vi "MemoryInitialize.vi"(8 "error in (no error)":errorcluster) -> (0 "error out":errorcluster)   [LabVIEW 2015]
uses:
  <vilib>/userdefined/High Color/IMAQdx.ctl
  [Global]CamNumber.vi
  [Global]ForCalCalculaton.vi
  [Global] ExtractedAnalizedImage.vi
  [Global] OperatorsImageTemplate2.vi
  [Global] ExtractedProcessImage.vi
  [Global] Coord.vi
  [Global] ExtractedImage.vi
  [Global] CameraSessionArray.vi
  [Global] CameraNameArray.vi
  [Global] Image.vi
  [Global] Image Overlay.vi
  [Global]Script Number.vi
  [Global]PatternMatchNumber.vi
  [Global] Template.vi
  [Global]SeqNumber.vi
  [Global]CalTemp.vi
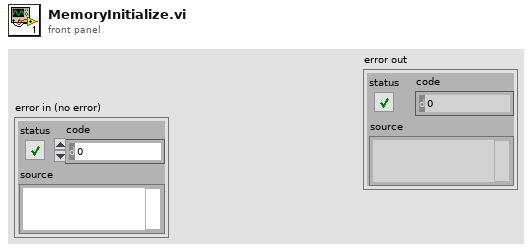
[diagram p1: front panel]
types:
  T1 = typedef "IMAQdx.ctl" = refnum<k21>
  T2 = typedef "IMAQ Image.ctl" = refnum<image>
  T3 = cluster{"Image Name":string, cluster{"Image Name":string, "New Image":T2}[]}
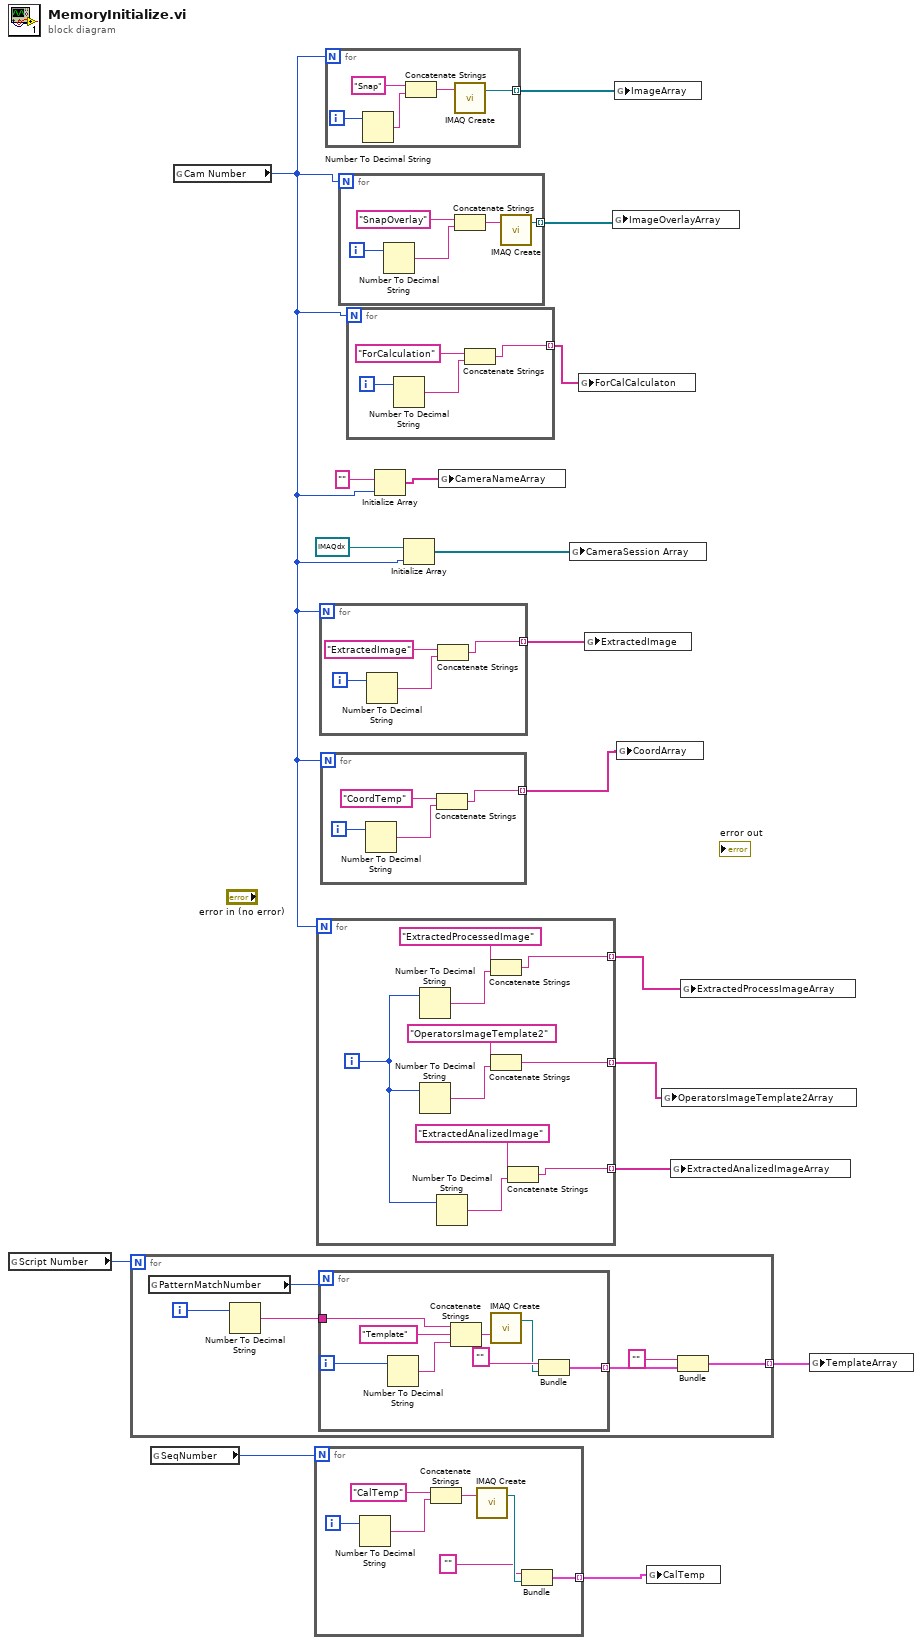
[diagram p0: block diagram]
diagram:
  n1 = global read "[Global]Script Number.vi" "Script Number"() -> (w3:i32)
  n2 = for {
    N: w3 -> [_]
    tunnel: [w18] -> w2 mode=indexing
    i -> [w20]
    n3 = global read "[Global]PatternMatchNumber.vi" "PatternMatchNumber"() -> (w21:i32)
    n4 = Number To Decimal String(number=w20) -> (decimal integer string=w19:string)  [unwired: 1 in]
    n5 = for {
      N: w21 -> [_]
      tunnel: [w29] -> w23 mode=indexing
      tunnel: w19 -> [w24]
      i -> [w27]
      n6 = Number To Decimal String(number=w27) -> (decimal integer string=w30:string)  [unwired: 1 in]
      n7 = Concatenate Strings(w24, "Template" ("Image Name"), w30) -> (w26:string)
      n8 = call "IMAQ Create"("Image Name"=w26) -> ("New Image"=w25:T2)  [unwired: 3 in, 2 out]
      n9 = Bundle("Image Name"="", "New Image"=w25) -> (w29:cluster{"Image Name":string, "New Image":T2})  [unwired: 1 in]
    }
    n10 = Bundle("Image Name"="", w23) -> (w18:T3)  [unwired: 1 in]
  }
  n11 = global read "[Global]SeqNumber.vi" "SeqNumber"() -> (w7:i32)
  n12 = global read "[Global]CamNumber.vi" "Cam Number"() -> (w5:i32)
  n13 = for {
    N: w7 -> [_]
    tunnel: [w32] -> w6 mode=indexing
    i -> [w37]
    n14 = Number To Decimal String(number=w37) -> (decimal integer string=w36:string)  [unwired: 1 in]
    n15 = Concatenate Strings("CalTemp" ("Image Name"), w36) -> (w35:string)
    n16 = call "IMAQ Create"("Image Name"=w35) -> ("New Image"=w34:T2)  [unwired: 3 in, 2 out]
    n17 = Bundle("Image Name"="", "New Image"=w34) -> (w32:cluster{"Image Name":string, "New Image":T2})  [unwired: 1 in]
  }
  n18 = for {
    N: w5 -> [_]
    tunnel: [w46] -> w10 mode=indexing
    tunnel: [w43] -> w9 mode=indexing
    tunnel: [w40] -> w8 mode=indexing
    i -> [w39]
    n19 = Number To Decimal String(number=w39) -> (decimal integer string=w47:string)  [unwired: 1 in]
    n20 = Number To Decimal String(number=w39) -> (decimal integer string=w45:string)  [unwired: 1 in]
    n21 = Number To Decimal String(number=w39) -> (decimal integer string=w41:string)  [unwired: 1 in]
    n22 = Concatenate Strings("ExtractedProcessedImage" ("Image Name"), w47) -> (w46:string)
    n23 = Concatenate Strings("OperatorsImageTemplate2" ("Image Name"), w45) -> (w43:string)
    n24 = Concatenate Strings("ExtractedAnalizedImage" ("Image Name"), w41) -> (w40:string)
  }
  n25 = for {
    N: w5 -> [_]
    tunnel: [w49] -> w11 mode=indexing
    i -> [w51]
    n26 = Number To Decimal String(number=w51) -> (decimal integer string=w50:string)  [unwired: 1 in]
    n27 = Concatenate Strings("ExtractedImage" ("Image Name"), w50) -> (w49:string)
  }
  n28 = for {
    N: w5 -> [_]
    tunnel: [w53] -> w1 mode=indexing
    i -> [w55]
    n29 = Number To Decimal String(number=w55) -> (decimal integer string=w54:string)  [unwired: 1 in]
    n30 = Concatenate Strings("CoordTemp" ("Image Name"), w54) -> (w53:string)
  }
  n31 = for {
    N: w5 -> [_]
    tunnel: [w57] -> w15 mode=indexing
    i -> [w61]
    n32 = Number To Decimal String(number=w61) -> (decimal integer string=w59:string)  [unwired: 1 in]
    n33 = Concatenate Strings("Snap", w59) -> (w58:string)
    n34 = call "IMAQ Create"("Image Name"=w58) -> ("New Image"=w57:T2)  [unwired: 3 in, 2 out]
  }
  n35 = for {
    N: w5 -> [_]
    tunnel: [w62] -> w14 mode=indexing
    i -> [w65]
    n36 = Number To Decimal String(number=w65) -> (decimal integer string=w64:string)  [unwired: 1 in]
    n37 = Concatenate Strings("SnapOverlay" ("Image Name"), w64) -> (w63:string)
    n38 = call "IMAQ Create"("Image Name"=w63) -> ("New Image"=w62:T2)  [unwired: 3 in, 2 out]
  }
  n39 = for {
    N: w5 -> [_]
    tunnel: [w67] -> w4 mode=indexing
    i -> [w69]
    n40 = Number To Decimal String(number=w69) -> (decimal integer string=w68:string)  [unwired: 1 in]
    n41 = Concatenate Strings("ForCalculation" ("Image Name"), w68) -> (w67:string)
  }
  n42 = Initialize Array("", w5) -> (w12:string[])
  n43 = Initialize Array(T1 refnum ("Session Out"), w5) -> (w16:T1[])
  n44 = global write "[Global] CameraNameArray.vi" "CameraNameArray"(w12) -> ()
  n45 = global write "[Global] CameraSessionArray.vi" "CameraSession Array"(w16) -> ()
  n46 = global write "[Global]ForCalCalculaton.vi" "ForCalCalculaton"(w4) -> ()
  n47 = global write "[Global] ExtractedImage.vi" "ExtractedImage"(w11) -> ()
  n48 = global write "[Global] Image Overlay.vi" "ImageOverlayArray"(w14) -> ()
  n49 = global write "[Global] Image.vi" "ImageArray"(w15) -> ()
  n50 = global write "[Global] Coord.vi" "CoordArray"(w1) -> ()
  n51 = global write "[Global]CalTemp.vi" "CalTemp"(w6) -> ()
  n52 = global write "[Global] OperatorsImageTemplate2.vi" "OperatorsImageTemplate2Array"(w9) -> ()
  n53 = global write "[Global] ExtractedAnalizedImage.vi" "ExtractedAnalizedImageArray"(w8) -> ()
  n54 = global write "[Global] ExtractedProcessImage.vi" "ExtractedProcessImageArray"(w10) -> ()
  n55 = global write "[Global] Template.vi" "TemplateArray"(w2) -> ()
